vi "LC Panel Initial.vi"(8 "error in (no error)":errorcluster caption="Error In") -> (0 "error out":errorcluster caption="Error Out")   [LabVIEW 2020]
uses:
  LC Single Control Information.ctl
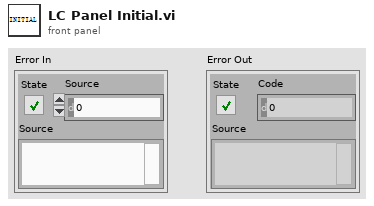
[diagram p1: front panel]
types:
  T1 = typedef "LC Single Control Information.ctl" = cluster{"VI Path":string, "VI Name":string, "Control Name":string, "Property Type":string, "Language":string, "Content":string}
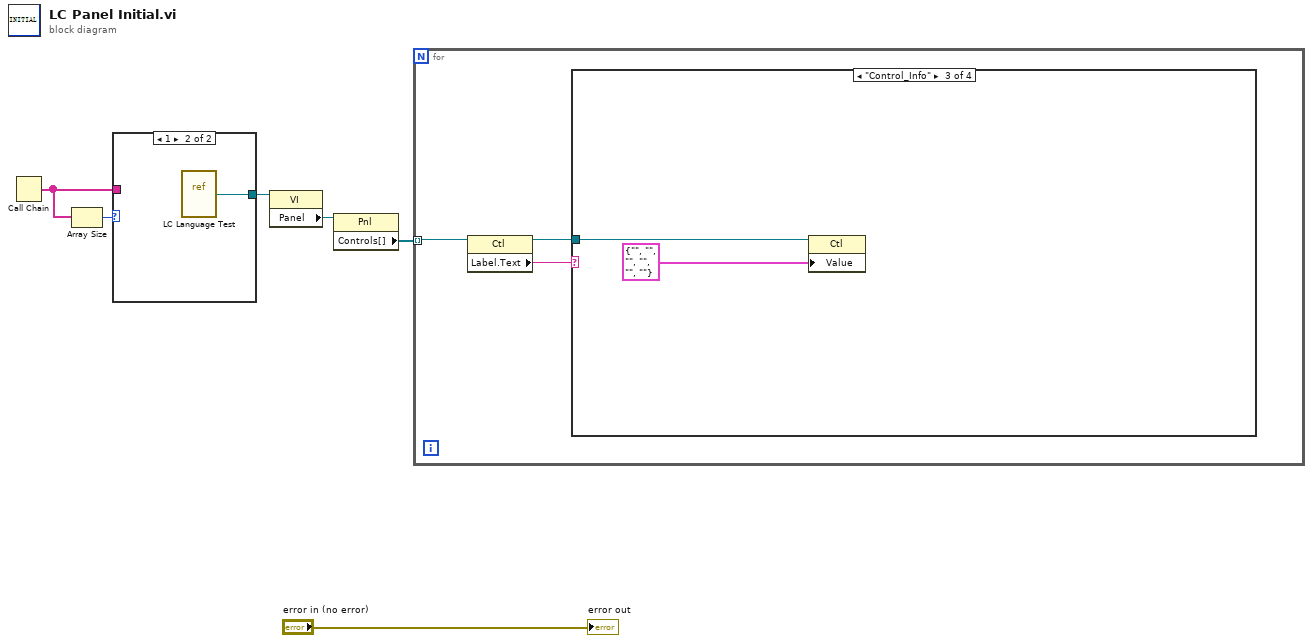
[diagram p0: block diagram]
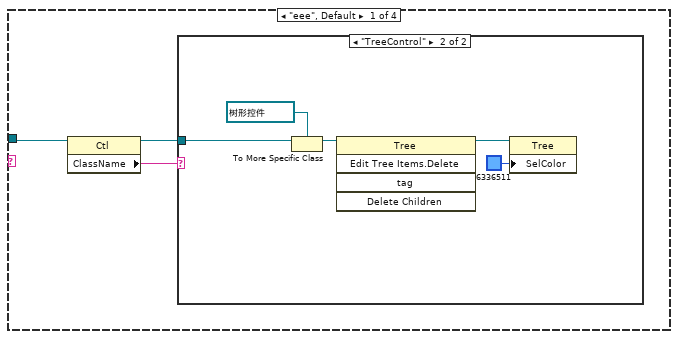
[diagram p2: hidden frame]
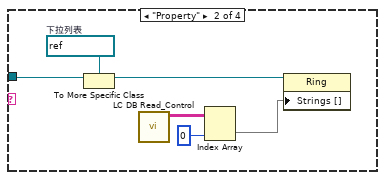
[diagram p4: hidden frame]
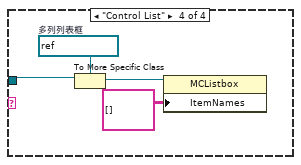
[diagram p5: hidden frame]
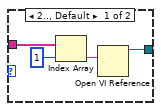
[diagram p6: hidden frame]
diagram:
  n1 = Call Chain() -> (call chain=w3:string[])
  n2 = Array Size(array=w3) -> (size(s)=w4:i32)
  n3 = case shown="1" w4 {
    tunnel: [w8 w11] -> w1
    tunnel: w3 -> [w7 _]
    frame 2.., Default {
      n4 = Index Array(array=w7, index=1 ("索引")) -> (element=w9:string)
      n5 = Open VI Reference(vi path=w9) -> (vi reference=w8:refnum<vi>)  [unwired: 5 in, 1 out]
    }
    frame 1 {
      n6 = vi-ref "LC Language Test.vi"() -> (w11:refnum<vi>)
    }
  }
  n7 = property class="VI"(reference=w1) -> ("Panel"=w2:refnum<vi>)  [unwired: 1 in, 2 out]
  n8 = property class="Pnl"(reference=w2) -> ("Controls[]"=w5:refnum<vi>[])  [unwired: 1 in, 2 out]
  n9 = for {
    tunnel: w5 -> [w14] mode=indexing
    n10 = property class="Ctl"(reference=w14) -> (reference out=w12:refnum<vi>, "Label.Text"=w13:string)  [unwired: 1 in, 1 out]
    n11 = case shown="\"Control_Info\"" w13 {
      tunnel: w12 -> [w17 w28 w30 w34]
      frame "eee", Default {
        n12 = property class="Ctl"(reference=w17) -> (reference out=w15:refnum<vi>, "ClassName"=w16:string)  [unwired: 1 in, 1 out]
        n13 = case shown="\"TreeControl\"" w16 {
          tunnel: w15 -> [_ w20]
          frame "假", Default {
          }
          frame "TreeControl" {
            n14 = To More Specific Class(target class=refnum<vi> refnum ("Control Path"), reference=w20) -> (specific class reference=w22:refnum<vi>)  [unwired: 1 in, 1 out]
            n15 = invoke class="Tree" method="Edit Tree Items.Delete"(reference=w22) -> (reference out=w19:refnum<vi>)  [unwired: 4 in, 4 out]
            n16 = property class="Tree"(reference=w19, "SelColor"=u32 6336511 ("选择颜色")) -> ()  [unwired: 1 in, 2 out]
          }
        }
      }
      frame "Property" {
        w27 = refnum<vi> refnum  # 下拉列表
        n17 = To More Specific Class(target class=w27, reference=w28) -> (specific class reference=w26:refnum<vi>)  [unwired: 1 in, 1 out]
        n18 = call "LC DB Read_Control.vi"() -> ("Data"=w25:string[][])  [unwired: 10 in, 1 out]
        n19 = Index Array(array=w25, index (col)=0 ("禁用的索引 (列)")) -> (element=w23:string[])  [unwired: 1 in]
        n20 = property class="Ring"(reference=w26, "Strings []"=w23) -> ()  [unwired: 1 in, 2 out]
      }
      frame "Control_Info" {
        n21 = property class="Ctl"(reference=w30, "Value"=T1 {"VI Path"="", "VI Name"="", "Control Name"="", "Property Type"="", "Language"="", "Content"=""} ("Control_Info")) -> ()  [unwired: 1 in, 2 out]
      }
      frame "Control List" {
        w33 = refnum<vi> refnum  # 多列列表框
        n22 = To More Specific Class(target class=w33, reference=w34) -> (specific class reference=w32:refnum<vi>)  [unwired: 1 in, 1 out]
        n23 = property class="MCListbox"(reference=w32, "ItemNames"=string[][] [] ("项名")) -> ()  [unwired: 1 in, 2 out]
      }
    }
  }
  "error out" <- "error in (no error)"
